vi "Toggle Annotation Shown.vi"(8 "error in (no error)":errorcluster, 11 "FSM.Edge in":refnum<class "FSM.Edge.lvclass">) -> (0 "error out":errorcluster, 3 "FSM.Edge out":refnum<class "FSM.Edge.lvclass">)   [LabVIEW 2015, in "FSM.Edge.lvclass"]
uses:
  FSM.Edge.lvclass
  FSM.Edge.lvclass/FSM.Edge.ctl
  FSM.Annotation/FSM.Annotation.lvclass/FSM.Annotation.ctl
  FSM.Annotation/Read Show.vi
  FSM.Annotation/Write Show.vi
  FSM.Annotation/FSM.Annotation.lvclass
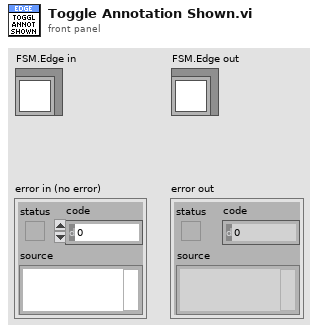
[diagram p1: front panel]
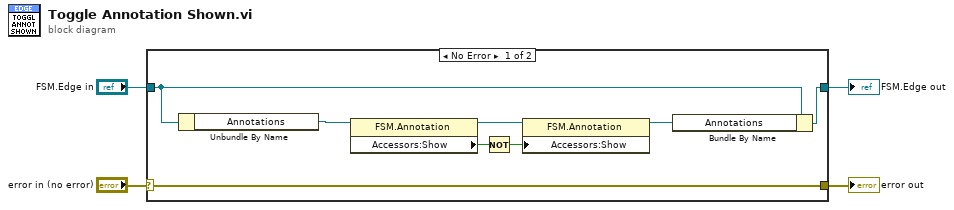
[diagram p0: block diagram]
diagram:
  n1 = case shown="No Error" "error in (no error)" {
    selector: "error in (no error)" -> [w12 w14]
    tunnel: [w12 w14] -> w3
    tunnel: [w7 w13] -> w1
    tunnel: "FSM.Edge in" -> [w11 w13]
    frame No Error {
      n2 = Unbundle By Name(w11) -> ("Annotations"=w10:refnum<class "FSM.Annotation.lvclass">)
      n3 = property class="FSM.Annotation"(reference=w10) -> (reference out=w8:refnum<class "FSM.Annotation.lvclass">, "Accessors:Show"=w9:bool)  [unwired: 1 in, 1 out]
      n4 = Not(x=w9) -> (.not. x?=w5:bool)
      n5 = property class="FSM.Annotation"(reference=w8, "Accessors:Show"=w5) -> (reference out=w6:refnum<class "FSM.Annotation.lvclass">)  [unwired: 1 in, 1 out]
      n6 = Bundle By Name(cluster=w11, "Annotations"=w6) -> (w7:refnum<class "FSM.Edge.lvclass">)
    }
    frame Error {
    }
  }
  "error out" <- w3
  "FSM.Edge out" <- w1
